vi "Return to Current.vi"(8 "error in":errorcluster, 10 "Speed(mm/s)":dbl=50.0, 11 "Gantry in":refnum<class "Gantry Class.lvclass">) -> (0 "error out":errorcluster, 3 "Gantry out":refnum<class "Gantry Class.lvclass">)   [LabVIEW 2011, in "Gantry Class.lvclass"]
uses:
  Gantry Class.lvclass
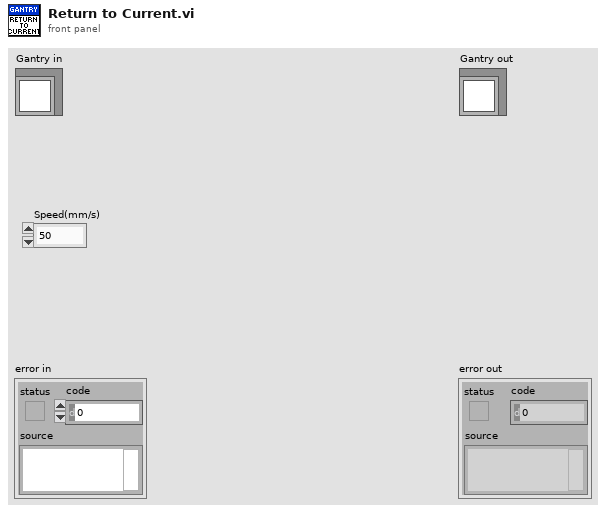
[diagram p1: front panel]
types:
  T1 = typedef "Named Position.ctl" = enum16{"home", "module_chuck_0", "module_chuck_1", "module_chuck_2", "module_chuck_3", "module_chuck_4", "glue_reservoir_chuck", "stamp_tool_chuck", "weight_tool_chuck", "needle_calibration", "tool_rack_pos_0_in", "tool_rack_pos_0_out", "tool_rack_pos_1_in", "tool_rack_pos_1_out", "tool_rack_pos_2_in", "tool_rack_pos_2_out", "front_load_position"}
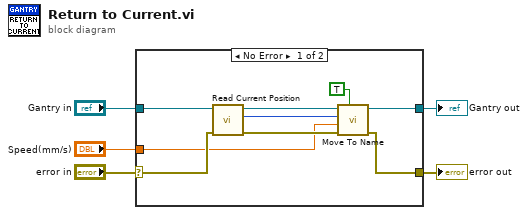
[diagram p0: block diagram]
diagram:
  n1 = case shown="No Error" "error in" {
    selector: "error in" -> [w11 w16]
    tunnel: [w10 w16] -> w4
    tunnel: [w6 w15] -> w2
    tunnel: "Gantry in" -> [w7 w15]
    tunnel: "Speed(mm/s)" -> [w9 _]
    frame No Error {
      n2 = call-dynamic "Read Current Position.vi"("error in"=w11, "Gantry in"=w7) -> ("error out"=w12:errorcluster, "Current Position"=w13:T1, "Gantry out"=w14:refnum<class "Gantry Class.lvclass">)  [unwired: 7 in]
      n3 = call-dynamic "Move To Name.vi"("Move if Same"=TRUE, "error in"=w12, "Speed(mm/s)"=w9, "Destination"=w13, "Gantry in"=w14) -> ("error out"=w10:errorcluster, "Gantry out"=w6:refnum<class "Gantry Class.lvclass">)  [unwired: 5 in]
    }
    frame Error {
    }
  }
  "error out" <- w4
  "Gantry out" <- w2
